vi "ClearFaults.vi"(11 "class data in":refnum<class "AbruptChange.lvclass">) -> (3 "class data out":refnum<class "AbruptChange.lvclass">)   [LabVIEW 2019, in "AbruptChange.lvclass"]
uses:
  AbruptChange.lvclass
  AbruptChange.lvclass/AbruptChange.ctl
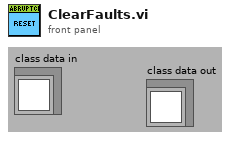
[diagram p1: front panel]
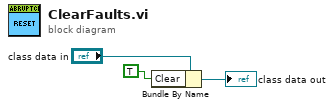
[diagram p0: block diagram]
diagram:
  n1 = Bundle By Name(cluster="class data in", "Clear"=TRUE ("Status")) -> (→"class data out":refnum<class "AbruptChange.lvclass">)
